vi "Release Stream.vi"(8 "error in (no error)":errorcluster, 10 "force destroy? (F)":bool, 11 "stream in":refnum<queue>) -> (0 "error out":errorcluster, 3 "remaining elements":T1[](array[typedef]))   [LabVIEW 2014]
uses:
  Action/Action.ctl
  Action/Action Name.ctl
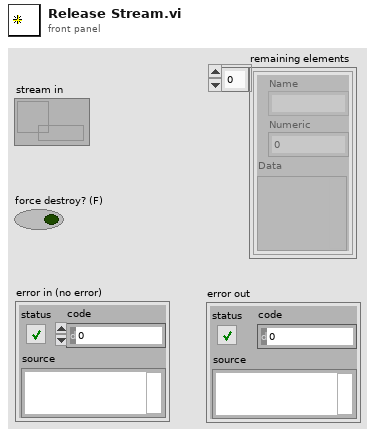
[diagram p1: front panel]
types:
  T1 = typedef "Action.ctl" = cluster{"Name":T2, "Numeric":i32, "Data":variant}
  T2 = typedef "Action Name.ctl" = enum16{""}
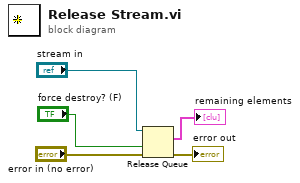
[diagram p0: block diagram]
diagram:
  n1 = Release Queue(queue="stream in", force destroy? (F)="force destroy? (F)", error in (no error)="error in (no error)") -> (remaining elements=→"remaining elements":T1[], error out=→"error out":errorcluster)  [unwired: 1 out]
